vi "DataLog Log Info.vi"(0 "tag log directory":path, 11 "error in (no error)":errorcluster) -> (4 "dup tag log directory":path, 8 "size":dbl, 10 "start time":dbl, 15 "error out":errorcluster)   [LabVIEW 2012]
doc: "Returns the log size, that is, the number of values (numbers or strings) contained in the tag's log. Since, on writing, logs are only appended to, this equals the write index. A double is used because it can represent very large integers without overflowing or rounding. In addition, the start time, that is, the timestamp of the first logged point is returned. When the log is empty, the start time is set to NaN."
uses:
  private/glb_DataLog MCVD.vi
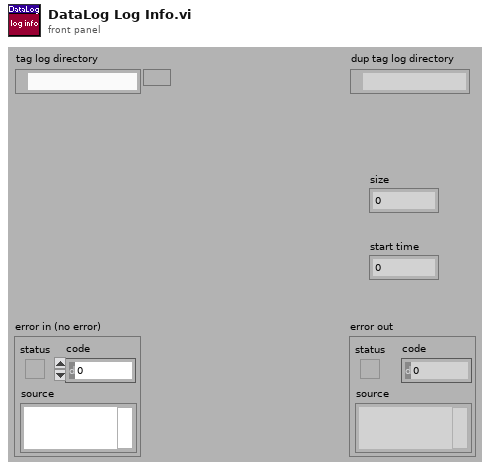
[diagram p1: front panel]
types:
  T1 = enum16{"read/write", "read-only", "write-only", "write-only (truncate)"}
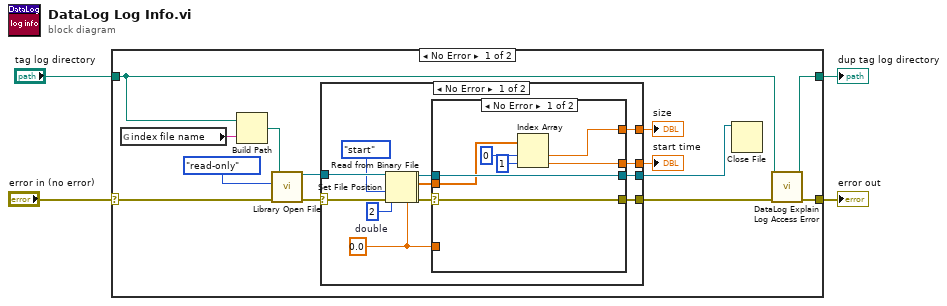
[diagram p0: block diagram]
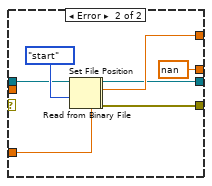
[diagram p2: hidden frame]
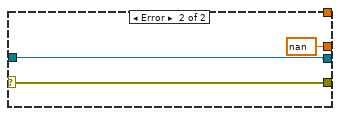
[diagram p3: hidden frame]
diagram:
  n1 = case shown="No Error" "error in (no error)" {
    selector: "error in (no error)" -> [w15 w52]
    tunnel: [w10 w52] -> w4
    tunnel: "tag log directory" -> [w8 w51]
    tunnel: [w9 w51] -> w1
    frame No Error {
      n2 = global read "glb_DataLog MCVD.vi" "index file name"() -> (w17:string)
      n3 = Build Path(base path=w8, name or relative path=w17) -> (appended path=w13:path)
      n4 = call "Library Open File.vi"("error in (no error)"=w15, "open mode (read/write)"=T1."read-only" ("open mode (0)"), "file path"=w13) -> ("error out"=w7:errorcluster, "refnum"=w12:refnum<file>)  [unwired: 3 in]
      n5 = case shown="No Error" w7 {
        selector: w7 -> [w29 w49]
        tunnel: [w21 w50] -> w16
        tunnel: w12 -> [w31 w50]
        tunnel: [w26 w49] -> w11
        tunnel: [w22 _] -> w6
        tunnel: [w20 nan ("double")] -> w5
        frame No Error {
          w23 = 0.0  # double
          n6 = Set File Position(refnum=w31, from (0:start)=enum16{"start", "end", "current"}."start" ("pos mode (0:2)"), error in=w29) -> (refnum out=w19:refnum<file>, error out=w18:errorcluster)  [unwired: 1 in]
          n7 = Read from Binary File(5:w23, 8:w18, 10:2 ("count"), 11:w19) -> (0:w27:errorcluster, 2:w25:dbl[], 3:w24:refnum<file>)  [unwired: 2 in, 1 out]
          n8 = case shown="No Error" w27 {
            selector: w27 -> [w38 _]
            tunnel: [w38 w43] -> w26
            tunnel: w25 -> [w36 _]
            tunnel: w24 -> [w37 w46]
            tunnel: w23 -> [_ w45]
            tunnel: [w32 w44] -> w22
            tunnel: [w37 w42] -> w21
            tunnel: [w33 nan ("double")] -> w20
            frame No Error {
              n9 = Index Array(array=w36, index #1=0 ("index"), index #2=1 ("index")) -> (element #1=w32:dbl, element #2=w33:dbl)
            }
            frame Error {
              n10 = Set File Position(refnum=w46, from (0:start)=enum16{"start", "end", "current"}."start" ("pos mode (0:2)")) -> (refnum out=w40:refnum<file>, error out=w39:errorcluster)  [unwired: 2 in]
              n11 = Read from Binary File(5:w45, 8:w39, 11:w40) -> (0:w43:errorcluster, 2:w44:dbl, 3:w42:refnum<file>)  [unwired: 3 in, 1 out]
            }
          }
        }
        frame Error {
        }
      }
      "size" <- w6
      "start time" <- w5
      n12 = Close File(refnum=w16) -> ()  [unwired: 1 in, 2 out]
      n13 = call "DataLog Explain Log Access Error.vi"("tag log directory"=w8, "error in"=w11) -> ("dup tag log directory"=w9:path, "error out"=w10:errorcluster)  [unwired: 12 in]
    }
    frame Error {
    }
  }
  "error out" <- w4
  "dup tag log directory" <- w1
